vi "IQ_Data_Processing.vi"(0 "file name":string, 2 "WFM Capture Response":T1, 3 "error in":errorcluster) -> (1 "gRPC error_status":i32, 4 "gRPC error_message":string, 5 "FFT Mag XY":cluster{"X":dbl[], "Y":dbl[]}[](array[cluster]), 6 "IQ XY":cluster{"X":dbl[], "Y":dbl[]}[](array[cluster]), 7 "error out":errorcluster)   [LabVIEW 2024]
uses:
  RPC Messages/rfcontrol_RFDCCaptureWaveformResponse.ctl
  FlexSDR_gRPC_client.lvlib
panel:
  out "Error Out":errorcluster
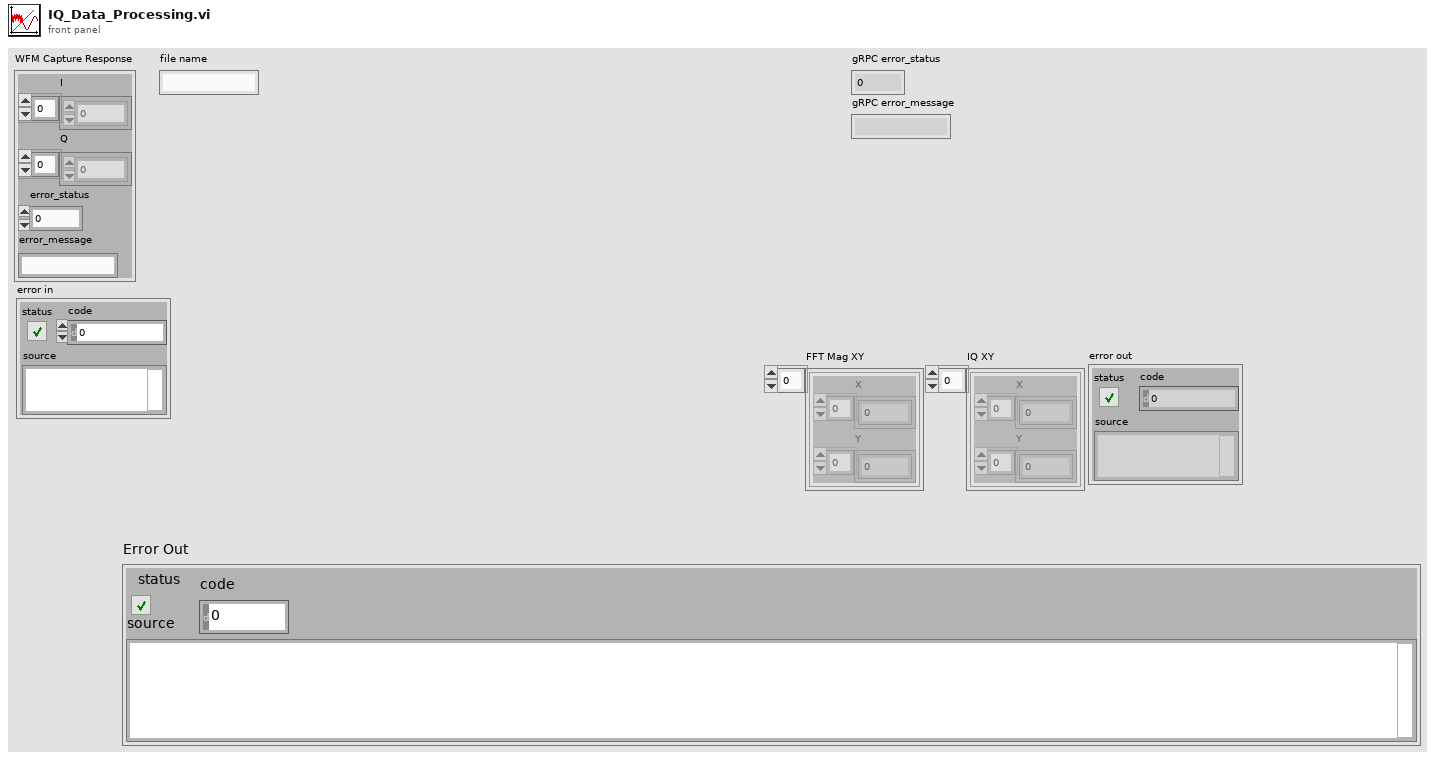
[diagram p1: front panel]
types:
  T1 = typedef "FlexSDR_gRPC_client.lvlib/rfcontrol_RFDCCaptureWaveformResponse.ctl" = cluster{"I":dbl[], "Q":dbl[], "error_status":i32, "error_message":string}
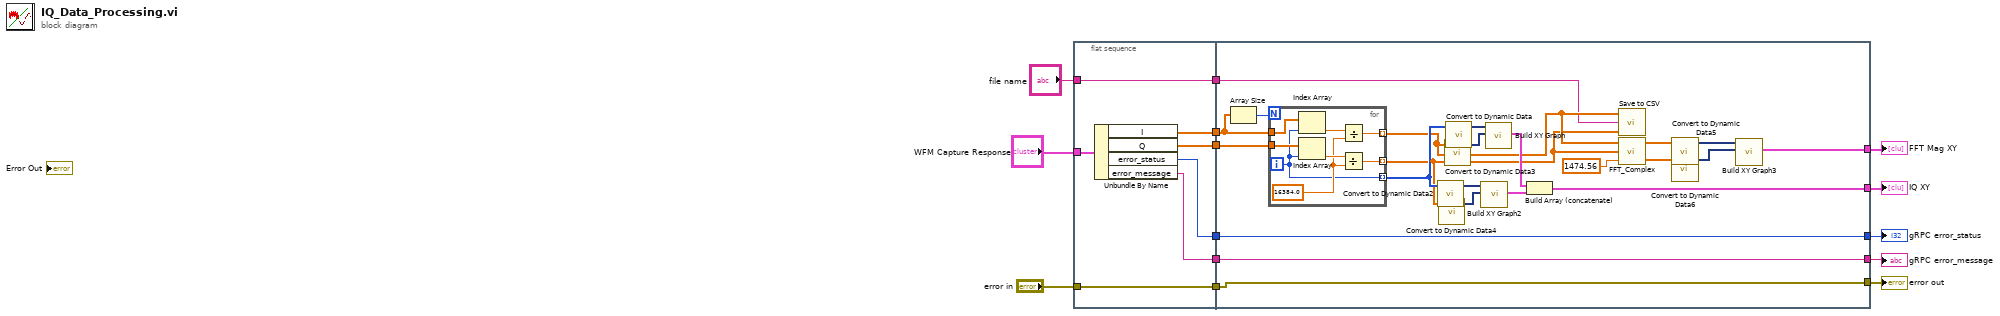
[diagram p0: block diagram]
diagram:
  n1 = flat-sequence {
    tunnel: "WFM Capture Response" -> [w21]
    tunnel: [w20] -> w14
    tunnel: [w19] -> w13
    tunnel: "file name" -> [w18]
    tunnel: [w18] -> w11
    tunnel: [w17] -> w10
    tunnel: [w16] -> w9
    tunnel: "error in" -> [w15]
    tunnel: [w15] -> w7
    tunnel: w14 -> [w42]
    tunnel: w13 -> [w43]
    tunnel: w11 -> [w27]
    tunnel: w10 -> [w25]
    tunnel: w9 -> [w26]
    tunnel: [w26] -> w4
    tunnel: [w25] -> w3
    tunnel: [w24] -> w5
    tunnel: [w23] -> w6
    tunnel: w7 -> [w22]
    tunnel: [w22] -> w2
    frame #0 {
      n2 = Unbundle By Name(w21) -> ("I"=w19:dbl[], "Q"=w20:dbl[], "error_status"=w16:i32, "error_message"=w17:string)
    }
    frame #1 {
      n3 = Array Size(array=w43) -> (size(s)=w44:i32)
      n4 = for {
        N: w44 -> [_]
        tunnel: w43 -> [w52]
        tunnel: w42 -> [w51]
        tunnel: [w47] -> w33 mode=indexing
        tunnel: [w46] -> w32 mode=indexing
        tunnel: [w45] -> w40 mode=indexing
        i -> [w45]
        w48 = 16384.0 ("y")
        n5 = Index Array(array=w52, index=w45) -> (element=w49:dbl)
        n6 = Index Array(array=w51, index=w45) -> (element=w50:dbl)
        n7 = Divide(x=w50, y=w48) -> (x/y=w46:dbl)
        n8 = Divide(x=w49, y=w48) -> (x/y=w47:dbl)
      }
      n9 = call "Convert to Dynamic Data2"("Array"=w40) -> ("Dynamic Data Type"=w39:dynamicdata)  [unwired: 3 in]
      n10 = call "Convert to Dynamic Data4"("Array"=w32) -> ("Dynamic Data Type"=w37:dynamicdata)  [unwired: 3 in]
      n11 = call "Convert to Dynamic Data3"("Array"=w33) -> ("Dynamic Data Type"=w38:dynamicdata)  [unwired: 3 in]
      n12 = call "Convert to Dynamic Data"("Array"=w40) -> ("Dynamic Data Type"=w41:dynamicdata)  [unwired: 3 in]
      n13 = call "Build XY Graph2"("Y Input"=w37, "X Input"=w39) -> ("XY Graph"=w35:cluster{"X":dbl[], "Y":dbl[]}[])  [unwired: 8 in, 1 out]
      n14 = call "Build XY Graph"("Y Input"=w38, "X Input"=w41) -> ("XY Graph"=w36:cluster{"X":dbl[], "Y":dbl[]}[])  [unwired: 8 in, 1 out]
      n15 = Build Array (concatenate)(w36, w35) -> (w24:cluster{"X":dbl[], "Y":dbl[]}[])
      n16 = call "Save to CSV.vi"("Q"=w32, "file name"=w27, "I"=w33) -> ()  [unwired: 1 in]
      n17 = call "FFT_Complex.vi"("Fs"=1474.56, "Q"=w32, "I"=w33) -> ("FFT Mag"=w29:dbl[], "FFT Freqs"=w31:dbl[])  [unwired: 1 in]
      n18 = call "Convert to Dynamic Data5"("Array"=w31) -> ("Dynamic Data Type"=w30:dynamicdata)  [unwired: 3 in]
      n19 = call "Convert to Dynamic Data6"("Array"=w29) -> ("Dynamic Data Type"=w28:dynamicdata)  [unwired: 3 in]
      n20 = call "Build XY Graph3"("Y Input"=w28, "X Input"=w30) -> ("XY Graph"=w23:cluster{"X":dbl[], "Y":dbl[]}[])  [unwired: 8 in, 1 out]
    }
  }
  "FFT Mag XY" <- w6
  "IQ XY" <- w5
  "gRPC error_status" <- w4
  "gRPC error_message" <- w3
  "error out" <- w2
